vi "GEA2 Stop.vi"(0 "GEA2 Reference In":refnum<k24>, 11 "Error In":errorcluster) -> (15 "Error Out":errorcluster)   [LabVIEW 2023]
doc: "This VI accepts a GEA2 bus reference and closes it. This VI should be used to close any open GEA2 connections before shutting down an application that uses the GEA2 bus."
uses:
  D:/Common/LabVIEW GEA2 Toolkit/source/GEA3 DLL Source/GeaCommunication.dll
  source/GEA3 DLL Source/GeaCommunication.dll
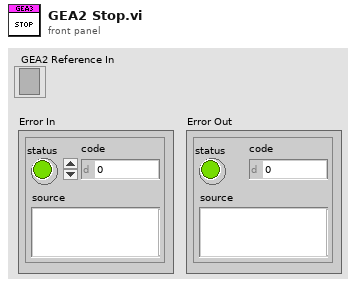
[diagram p1: front panel]
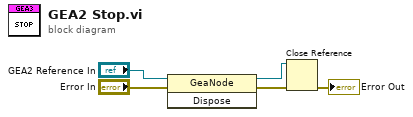
[diagram p0: block diagram]
diagram:
  n1 = invoke class="GeaNode" method="Dispose"(reference="GEA2 Reference In", error in="Error In") -> (reference out=w4:refnum<k24>, error out=w5:errorcluster)  [unwired: 1 in, 1 out]
  n2 = Close Reference(reference=w4, error in (no error)=w5) -> (error out=→"Error Out":errorcluster)
